vi "Read PressCoeff.vi"(8 "error in (no error)":errorcluster, 11 "BMP208 in":refnum<class "BMP208.lvclass">) -> (0 "error out":errorcluster, 2 "PressCoeff":T1, 3 "BMP208 out":refnum<class "BMP208.lvclass">)   [LabVIEW 2020, in "BMP208.lvclass"]
uses:
  BMP208.lvclass
  Controls/td_cluster_Press_Coeff.ctl
  BMP208.lvclass/BMP208.ctl
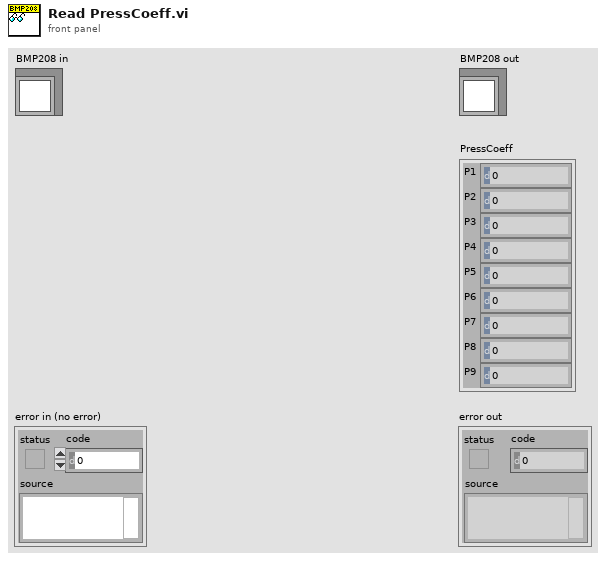
[diagram p1: front panel]
types:
  T1 = typedef "BMP208.lvclass/td_cluster_Press_Coeff.ctl" = cluster{"P1":u16, "P2":i16, "P3":i16, "P4":i16, "P5":i16, "P6":i16, "P7":i16, "P8":i16, "P9":i16}
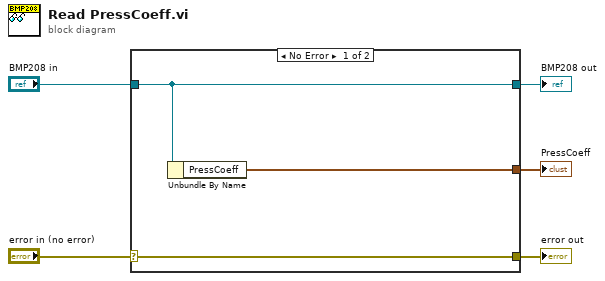
[diagram p0: block diagram]
diagram:
  n1 = case shown="No Error" "error in (no error)" {
    selector: "error in (no error)" -> [w8 w9]
    tunnel: [w8 w9] -> w4
    tunnel: [w7 w10] -> w2
    tunnel: "BMP208 in" -> [w7 w10]
    tunnel: [w6 _] -> w1
    frame No Error {
      n2 = Unbundle By Name(w7) -> ("PressCoeff"=w6:T1)
    }
    frame Error {
    }
  }
  "error out" <- w4
  "BMP208 out" <- w2
  "PressCoeff" <- w1
